vi "Modbus 32bit Number Combine.vi"(11 "Holding Registers":u16[](array[numeric])) -> (3 "Numeric":sgl)   [LabVIEW 2012]
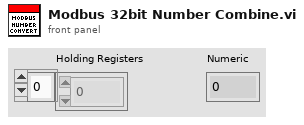
[diagram p1: front panel]
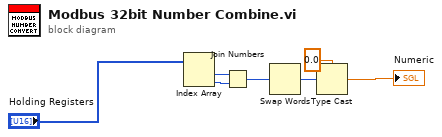
[diagram p0: block diagram]
diagram:
  n1 = Index Array(array="Holding Registers") -> (element #1=w4:u16, element #2=w5:u16)  [unwired: 2 in]
  n2 = Join Numbers(hi=w4, lo=w5) -> ((hi.lo)=w2:u32)
  n3 = Swap Words(1:w2) -> (0:w1:u32)
  n4 = Type Cast(type=sgl 0.0, x=w1) -> (*(type *) &x=→"Numeric":sgl)
